vi "波形数据的均值化2.vi"(0 "传感器灵敏度":dbl=1.0, 1 "传感器灵敏度 2":dbl=1.0, 2 "温度信号":waveform(dbl)[](graph), 4 "传感器灵敏度 3":dbl=1.0, 5 "传感器灵敏度 4":dbl=1.0, 14 "传感器灵敏度 5":dbl=1.0, 15 "传感器灵敏度 6":dbl=1.0, 18 "传感器灵敏度 7":dbl=1.0, 19 "传感器灵敏度 8":dbl=1.0) -> (6 "传感器与轴的距离":dbl, 7 "传感器与轴的距离 5":dbl, 8 "传感器与轴的距离 2":dbl, 9 "传感器与轴的距离 6":dbl, 10 "传感器与轴的距离 3":dbl, 11 "传感器与轴的距离 7":dbl, 12 "传感器与轴的距离 4":dbl, 13 "传感器与轴的距离 8":dbl, 16 "温度信号 3":waveform(dbl)[](graph))   [LabVIEW 2014]
panel:
  out "元素":i32
  out "大小":i32[](array[numeric])
  out "Array":dbl[][](array[numeric]) caption="数组"
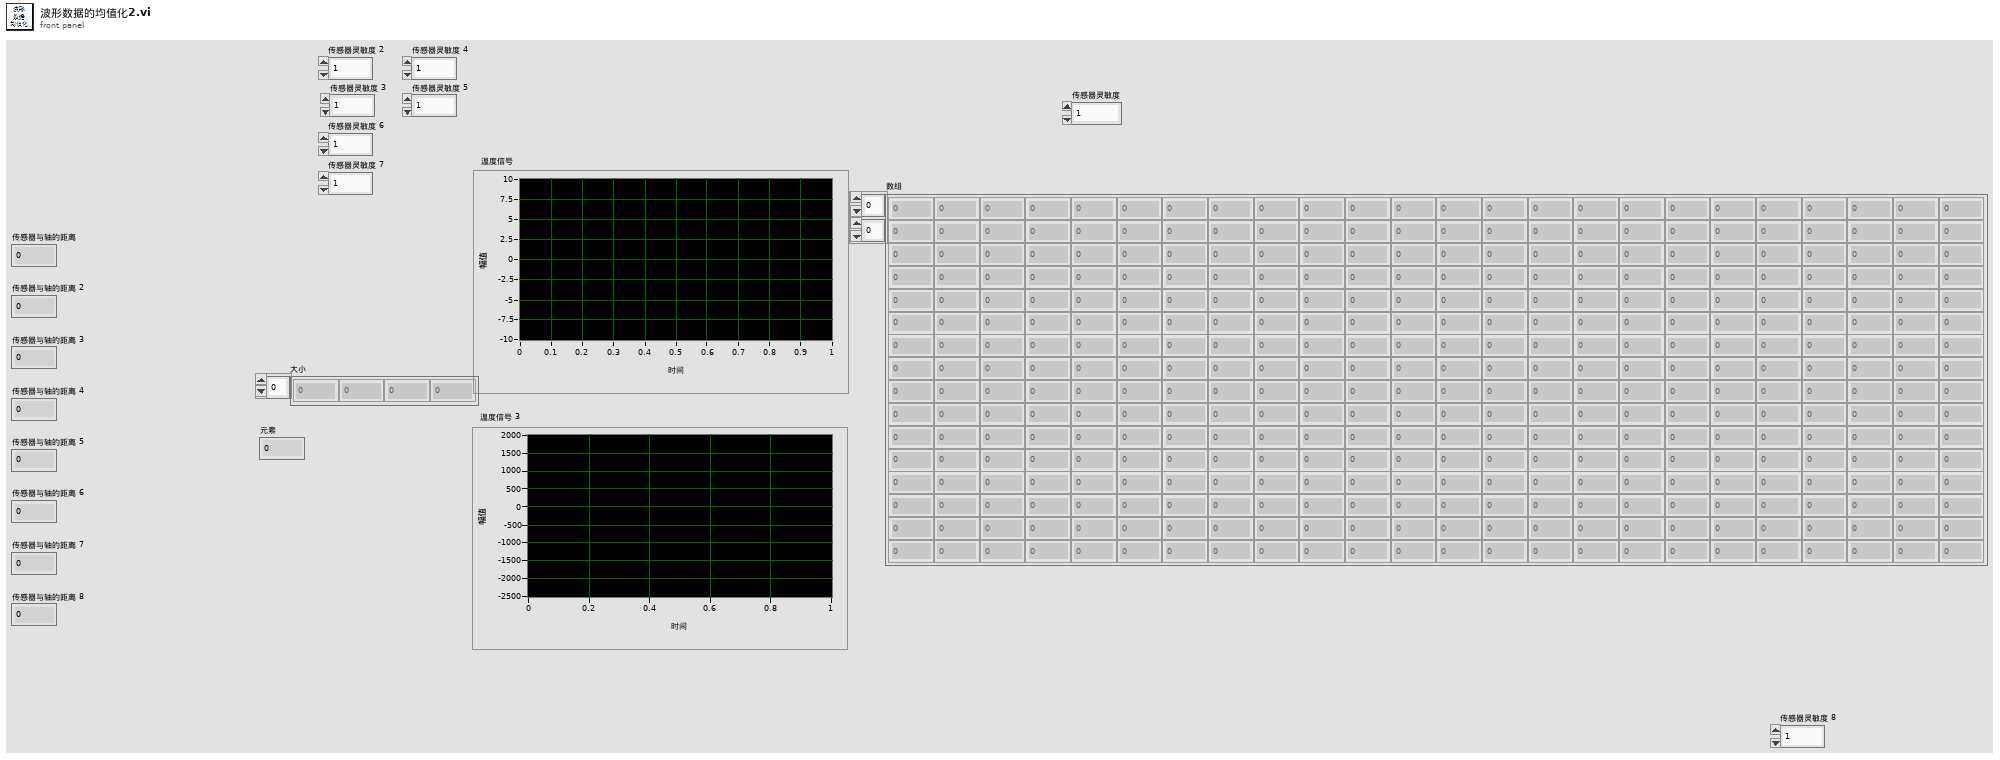
[diagram p1: front panel]
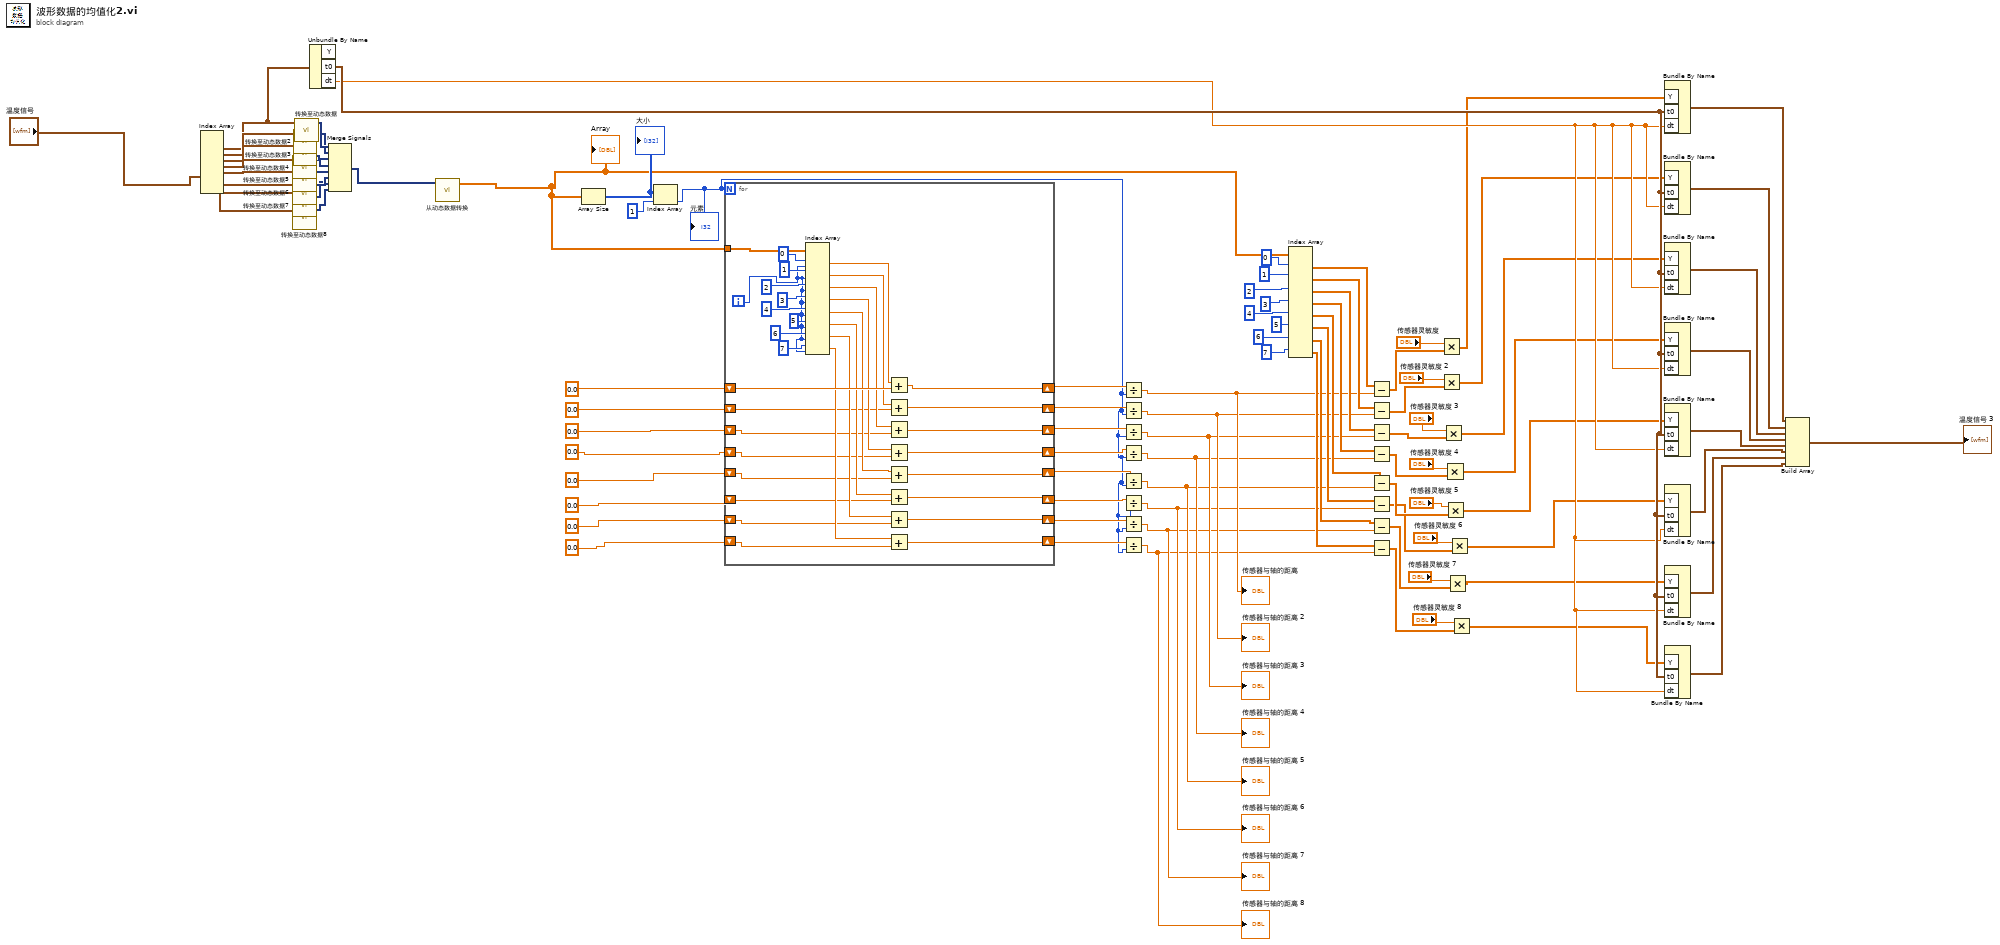
[diagram p0: block diagram]
diagram:
  n1 = Index Array(array="温度信号") -> (element #1=w46:waveform(dbl), element #2=w89:waveform(dbl), element #3=w88:waveform(dbl), element #4=w87:waveform(dbl), element #5=w86:waveform(dbl), element #6=w85:waveform(dbl), element #7=w84:waveform(dbl), element #8=w83:waveform(dbl))  [unwired: 8 in]
  n2 = call "转换至动态数据4"("Waveform"=w87) -> ("Dynamic Data Type"=w94:dynamicdata)  [unwired: 3 in]
  n3 = call "转换至动态数据5"("Waveform"=w86) -> ("Dynamic Data Type"=w93:dynamicdata)  [unwired: 3 in]
  n4 = call "转换至动态数据6"("Waveform"=w85) -> ("Dynamic Data Type"=w92:dynamicdata)  [unwired: 3 in]
  n5 = call "转换至动态数据7"("Waveform"=w84) -> ("Dynamic Data Type"=w91:dynamicdata)  [unwired: 3 in]
  n6 = call "转换至动态数据8"("Waveform"=w83) -> ("Dynamic Data Type"=w90:dynamicdata)  [unwired: 3 in]
  n7 = call "转换至动态数据2"("Waveform"=w89) -> ("Dynamic Data Type"=w96:dynamicdata)  [unwired: 3 in]
  n8 = call "转换至动态数据3"("Waveform"=w88) -> ("Dynamic Data Type"=w95:dynamicdata)  [unwired: 3 in]
  n9 = call "转换至动态数据"("Waveform"=w46) -> ("Dynamic Data Type"=w97:dynamicdata)  [unwired: 3 in]
  n10 = Unbundle By Name(w46) -> ("t0"=w45:timestamp, "dt"=w44:dbl)  [unwired: 1 out]
  n11 = Merge Signals(w97, w96, w95, w94, w93, w92, w91, w90) -> (w47:dynamicdata)
  n12 = call "从动态数据转换"("Dynamic Data Type"=w47) -> ("Array"=w25:dbl[][])  [unwired: 3 in]
  "Array" <- w25
  n13 = Array Size(array=w25) -> (size(s)=w50:i32[])
  "大小" <- w50
  n14 = Index Array(array=w50, index=1) -> (element=w49:i32)
  "元素" <- w49
  n15 = for {
    N: w49 -> [_]
    tunnel: w25 -> [w129]
    shift-right: [w105] -> w73
    shift-left: 0.0 -> [w121]
    shift-right: [w104] -> w72
    shift-left: 0.0 -> [w112]
    shift-right: [w103] -> w71
    shift-left: 0.0 -> [w111]
    shift-right: [w102] -> w70
    shift-left: 0.0 -> [w110]
    shift-right: [w101] -> w69
    shift-left: 0.0 -> [w109]
    shift-right: [w100] -> w68
    shift-left: 0.0 -> [w108]
    shift-right: [w99] -> w67
    shift-left: 0.0 -> [w107]
    shift-right: [w98] -> w66
    shift-left: 0.0 -> [w106]
    i -> [w122]
    n16 = Index Array(array=w129, index (row) #1=0 ("索引 (行)"), index (col) #1=w122, index (row) #2=1 ("索引 (行)"), index (col) #2=w122, index (row) #3=2 ("索引 (行)"), index (col) #3=w122, index (row) #4=3 ("索引 (行)"), index (col) #4=w122, index (row) #5=4 ("索引 (行)"), index (col) #5=w122, index (row) #6=5 ("索引 (行)"), index (col) #6=w122, index (row) #7=6 ("索引 (行)"), index (col) #7=w122, index (row) #8=7 ("索引 (行)"), index (col) #8=w122) -> (element #1=w120:dbl, element #2=w119:dbl, element #3=w118:dbl, element #4=w117:dbl, element #5=w116:dbl, element #6=w115:dbl, element #7=w114:dbl, element #8=w113:dbl)
    n17 = Add(x=w120, y=w121) -> (x+y=w105:dbl)
    n18 = Add(x=w119, y=w112) -> (x+y=w104:dbl)
    n19 = Add(x=w118, y=w111) -> (x+y=w103:dbl)
    n20 = Add(x=w117, y=w110) -> (x+y=w102:dbl)
    n21 = Add(x=w116, y=w109) -> (x+y=w101:dbl)
    n22 = Add(x=w115, y=w108) -> (x+y=w100:dbl)
    n23 = Add(x=w114, y=w107) -> (x+y=w99:dbl)
    n24 = Add(x=w113, y=w106) -> (x+y=w98:dbl)
  }
  n25 = Divide(x=w73, y=w49) -> (x/y=w34:dbl)
  "传感器与轴的距离" <- w34
  n26 = Divide(x=w72, y=w49) -> (x/y=w33:dbl)
  "传感器与轴的距离 2" <- w33
  n27 = Divide(x=w71, y=w49) -> (x/y=w32:dbl)
  "传感器与轴的距离 3" <- w32
  n28 = Divide(x=w70, y=w49) -> (x/y=w31:dbl)
  "传感器与轴的距离 4" <- w31
  n29 = Divide(x=w69, y=w49) -> (x/y=w30:dbl)
  "传感器与轴的距离 5" <- w30
  n30 = Divide(x=w68, y=w49) -> (x/y=w29:dbl)
  "传感器与轴的距离 6" <- w29
  n31 = Divide(x=w67, y=w49) -> (x/y=w28:dbl)
  "传感器与轴的距离 7" <- w28
  n32 = Divide(x=w66, y=w49) -> (x/y=w27:dbl)
  "传感器与轴的距离 8" <- w27
  n33 = Index Array(array=w25, index (row) #1=0 ("索引 (行)"), index (row) #2=1 ("索引 (行)"), index (row) #3=2 ("索引 (行)"), index (row) #4=3 ("索引 (行)"), index (row) #5=4 ("索引 (行)"), index (row) #6=5 ("索引 (行)"), index (row) #7=6 ("索引 (行)"), index (row) #8=7 ("索引 (行)")) -> (element #1=w26:dbl[], element #2=w57:dbl[], element #3=w56:dbl[], element #4=w55:dbl[], element #5=w54:dbl[], element #6=w53:dbl[], element #7=w52:dbl[], element #8=w51:dbl[])  [unwired: 8 in]
  n34 = Subtract(x=w26, y=w34) -> (x-y=w17:dbl[])
  n35 = Subtract(x=w57, y=w33) -> (x-y=w15:dbl[])
  n36 = Subtract(x=w56, y=w32) -> (x-y=w14:dbl[])
  n37 = Subtract(x=w55, y=w31) -> (x-y=w11:dbl[])
  n38 = Subtract(x=w54, y=w30) -> (x-y=w9:dbl[])
  n39 = Subtract(x=w53, y=w29) -> (x-y=w5:dbl[])
  n40 = Subtract(x=w52, y=w28) -> (x-y=w4:dbl[])
  n41 = Subtract(x=w51, y=w27) -> (x-y=w3:dbl[])
  n42 = Multiply(x="传感器灵敏度", y=w17) -> (x*y=w16:dbl[])
  n43 = Multiply(x="传感器灵敏度 2", y=w15) -> (x*y=w13:dbl[])
  n44 = Multiply(x="传感器灵敏度 3", y=w14) -> (x*y=w12:dbl[])
  n45 = Multiply(x="传感器灵敏度 4", y=w11) -> (x*y=w10:dbl[])
  n46 = Multiply(x="传感器灵敏度 5", y=w9) -> (x*y=w8:dbl[])
  n47 = Multiply(x="传感器灵敏度 7", y=w4) -> (x*y=w2:dbl[])
  n48 = Multiply(x="传感器灵敏度 6", y=w5) -> (x*y=w7:dbl[])
  n49 = Multiply(x="传感器灵敏度 8", y=w3) -> (x*y=w1:dbl[])
  n50 = Bundle By Name("Y"=w16, "t0"=w45, "dt"=w44) -> (w43:waveform(dbl))  [unwired: 1 in]
  n51 = Bundle By Name("Y"=w13, "t0"=w45, "dt"=w44) -> (w42:waveform(dbl))  [unwired: 1 in]
  n52 = Bundle By Name("Y"=w12, "t0"=w45, "dt"=w44) -> (w41:waveform(dbl))  [unwired: 1 in]
  n53 = Bundle By Name("Y"=w10, "t0"=w45, "dt"=w44) -> (w40:waveform(dbl))  [unwired: 1 in]
  n54 = Bundle By Name("Y"=w8, "t0"=w45, "dt"=w44) -> (w39:waveform(dbl))  [unwired: 1 in]
  n55 = Bundle By Name("Y"=w7, "t0"=w45, "dt"=w44) -> (w38:waveform(dbl))  [unwired: 1 in]
  n56 = Bundle By Name("Y"=w2, "t0"=w45, "dt"=w44) -> (w37:waveform(dbl))  [unwired: 1 in]
  n57 = Bundle By Name("Y"=w1, "t0"=w45, "dt"=w44) -> (w36:waveform(dbl))  [unwired: 1 in]
  n58 = Build Array(w43, w42, w41, w40, w39, w38, w37, w36) -> (→"温度信号 3":waveform(dbl)[])
